vi "mxwScript_Cmnd2Str_setDropArea.vi"(8 "error in (no error)":errorcluster, 11 "data":variant) -> (0 "error out":errorcluster, 3 "outputString":string)   [LabVIEW 2020]
uses:
  codeGenAPISupport.llb/cgAPI_mxwScript_DropArea.ctl
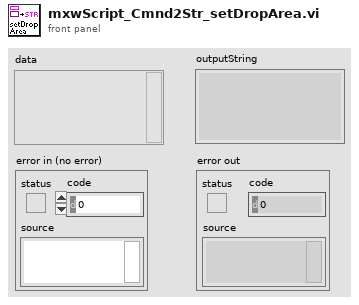
[diagram p1: front panel]
types:
  T1 = typedef "cgAPI_mxwScript_DropArea.ctl" = cluster{"XMax":i32, "XMin":i32, "YMax":i32, "YMin":i32, "XInc":i32, "YInc":i32}
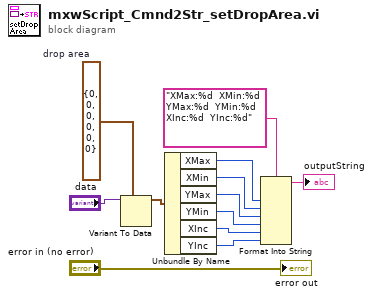
[diagram p0: block diagram]
diagram:
  w7 = T1 {"XMax"=0, "XMin"=0, "YMax"=0, "YMin"=0, "XInc"=0, "YInc"=0}  # drop area
  n1 = Variant To Data(type=w7, Variant="data") -> (data=w10:T1)  [unwired: 1 in, 1 out]
  n2 = Unbundle By Name(w10) -> ("XMax"=w5:i32, "XMin"=w4:i32, "YMax"=w3:i32, "YMin"=w2:i32, "XInc"=w1:i32, "YInc"=w6:i32)
  n3 = Format Into String(format string="XMax:%d  XMin:%d  YMax:%d  YMin:%d  XInc:%d  YInc:%d", w5, w4, w3, w2, w1, w6) -> (resulting string=→"outputString":string)  [unwired: 2 in, 1 out]
  "error out" <- "error in (no error)"
